vi "ex_createTdmTimeChannels.vi"(4 "error in (no error)":errorcluster, 5 "waveform":waveform(dbl), 6 "All Express Wave Attributes Plus":T1 {"dX" format="%.2f"; "X0" format="%<%X\n%x>T"; "Timestamp" format="%<%X\n%x>T"; "Start Timestamp" format="%<%X\n%x>T"}, 7 "Data object in":refnum<k20>) -> (0 "error out":errorcluster, 1 "Length":u32, 3 "Data object out":refnum<k20>)   [LabVIEW 2017]
uses:
  <vilib>/express/express shared/transition.llb/ex_WaveformAttribsPlus.ctl
  <vilib>/Platform/storage/lvStorage.llb/_wf_attributes.ctl
  <vilib>/Platform/storage/Storage.llb/__savePropTime.vi
  <vilib>/Platform/storage/Storage.llb/__loadPropRef.vi
  <vilib>/Platform/storage/Storage.llb/__loadPropTime.vi
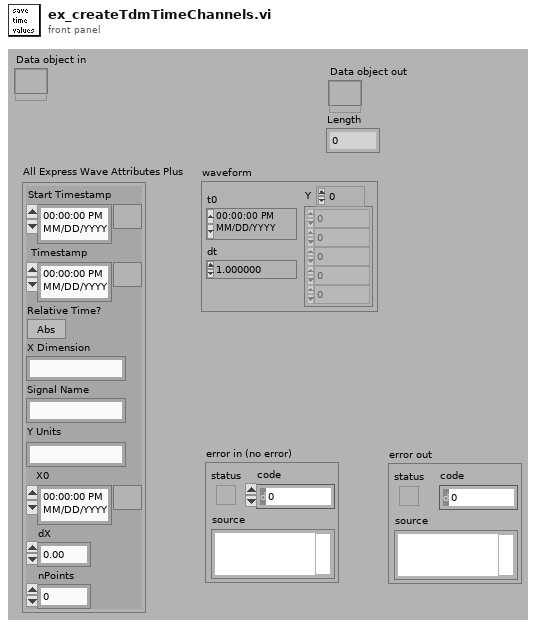
[diagram p1: front panel]
types:
  T1 = typedef "ex_WaveformAttribsPlus.ctl" = cluster{"Start Timestamp":timestamp, "Timestamp":timestamp, "Relative Time?":bool, "X Dimension":string, "Signal Name":string, "Y Units":string, "X0":timestamp, "dX":dbl, "nPoints":i32}
  T2 = typedef "_wf_attributes.ctl" = enum16{"t0", "dt", "X_Name", "X_Unit", "x0", "abs/rel", "nPoints", "file_timestamp", "xcolumns"}
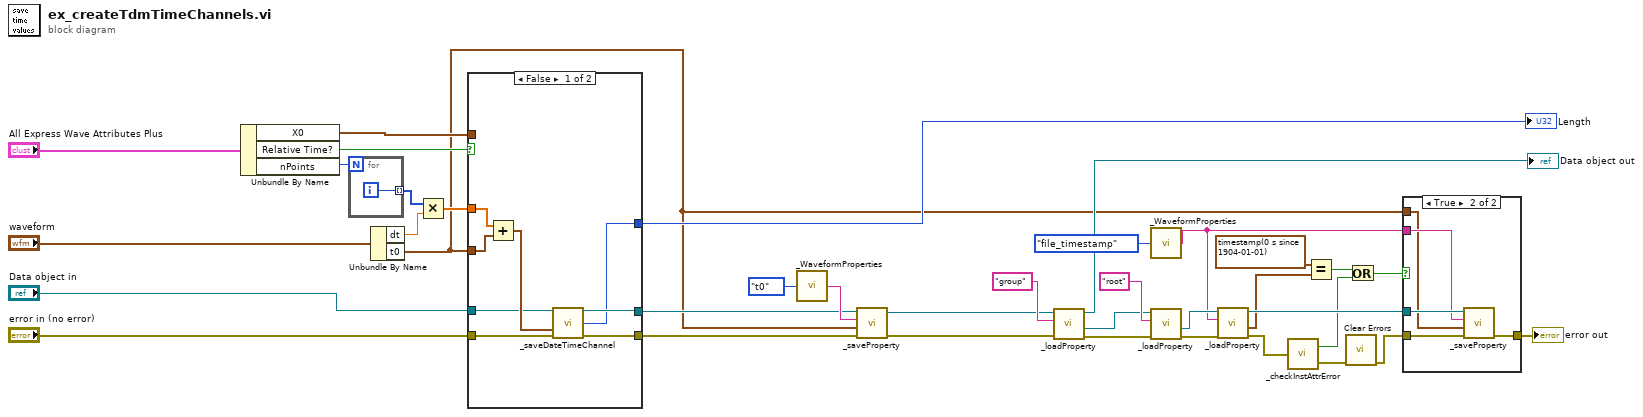
[diagram p0: block diagram]
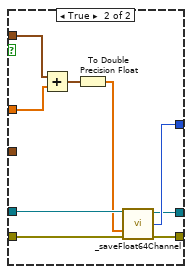
[diagram p3: hidden frame]
diagram:
  n1 = Unbundle By Name("All Express Wave Attributes Plus") -> ("X0"=w28:timestamp, "Relative Time?"=w31:bool, "nPoints"=w36:i32)
  n2 = for {
    N: w36 -> [_]
    tunnel: [w38] -> w33 mode=indexing
    i -> [w38]
  }
  n3 = Unbundle By Name("waveform") -> ("dt"=w32:dbl, "t0"=w3:timestamp)
  n4 = Multiply(x=w33, y=w32) -> (x*y=w30:dbl[])
  n5 = case shown="False" w31 {
    tunnel: [w45 w47] -> w5
    tunnel: "error in (no error)" -> [w46 w55]
    tunnel: w30 -> [w44 w52]
    tunnel: "Data object in" -> [w42 w54]
    tunnel: [w41 w48] -> w4
    tunnel: [w40 w49] -> w9
    tunnel: w28 -> [_ w53]
    tunnel: w3 -> [w39 _]
    frame False {
      n6 = Add(x=w44, y=w39) -> (x+y=w43:timestamp[])
      n7 = call <vilib>:"_saveDateTimeChannel.vi"("Data object in"=w42, "Values"=w43, "error in (no error)"=w46) -> ("Data object out"=w41:refnum<k20>, "Length"=w40:u32, "error out"=w45:errorcluster)  [unwired: 6 in, 4 out]
    }
    frame True {
      n8 = Add(x=w53, y=w52) -> (x+y=w51:timestamp[])
      n9 = To Double Precision Float(number=w51) -> (double precision float=w50:dbl[])
      n10 = call <vilib>:"_saveFloat64Channel.vi"("Data object in"=w54, "Values"=w50, "error in (no error)"=w55) -> ("Data object out"=w48:refnum<k20>, "Length"=w49:u32, "error out"=w47:errorcluster)  [unwired: 6 in, 4 out]
    }
  }
  "Length" <- w9
  n11 = call <vilib>:"_WaveformProperties.vi"("Property"=_wf_attributes."t0") -> ("Name"=w7:string)
  n12 = call-poly <vilib>:"_saveProperty.vi"("error in (no error)"=w5, "Value"=w3, "Property name"=w7, "storage refnum"=w4) -> ("error out"=w2:errorcluster, "dup storage refnum"=w1:refnum<k20>)  [unwired: 1 in, 5 out]
  n13 = call-poly <vilib>:"_loadProperty.vi"("error in (no error)"=w2, "Property name"="group" ("PropertyName"), "storage refnum"=w1) -> ("error out"=w26:errorcluster, "Value"=w16:refnum<k20>, "dup storage refnum"=→"Data object out":refnum<k20>)  [unwired: 6 out]
  n14 = call <vilib>:"_WaveformProperties.vi"("Property"=_wf_attributes."file_timestamp") -> ("Name"=w14:string)
  n15 = call-poly <vilib>:"_loadProperty.vi"("error in (no error)"=w26, "Property name"="root" ("PropertyName"), "storage refnum"=w16) -> ("error out"=w24:errorcluster, "Value"=w23:refnum<k20>)  [unwired: 7 out]
  n16 = call-poly <vilib>:"_loadProperty.vi"("error in (no error)"=w24, "Property name"=w14, "storage refnum"=w23) -> ("error out"=w13:errorcluster, "Value"=w20:timestamp, "dup storage refnum"=w22:refnum<k20>)  [unwired: 6 out]
  n17 = call <vilib>:"_checkInstAttrError.vi"("error in (no error)"=w13) -> ("Create?"=w11:bool, "error out"=w12:errorcluster)
  n18 = Equal?(x=timestamp(0 s since 1904-01-01), y=w20) -> (x = y?=w19:bool)
  n19 = call <vilib>:"Clear Errors.vi"("error in (no error)"=w12) -> ("error out"=w17:errorcluster)  [unwired: 1 in, 5 out]
  n20 = Or(x=w19, y=w11) -> (x .or. y?=w18:bool)
  n21 = case shown="True" w18 {
    tunnel: w22 -> [_ w61]
    tunnel: w14 -> [_ w60]
    tunnel: w3 -> [_ w59]
    tunnel: [w56 w58] -> w8
    tunnel: w17 -> [w56 w57]
    frame False {
    }
    frame True {
      n22 = call-poly <vilib>:"_saveProperty.vi"("error in (no error)"=w57, "Value"=w59, "Property name"=w60, "storage refnum"=w61) -> ("error out"=w58:errorcluster)  [unwired: 1 in, 6 out]
    }
  }
  "error out" <- w8
